vi "反馈节点 1.vi"() -> ()   [LabVIEW 2023]
panel:
  out "compile or load":dbl[](array[numeric])
  out "first call":dbl[](array[numeric])
  out "Array":i32[](array[numeric])
  # "反馈节点 1"
  # "例子 1"
  # "运行 两次以后"
  # "反馈节点 如果初始值 设为 compile or load \n那么 feedback node value will keep last value"
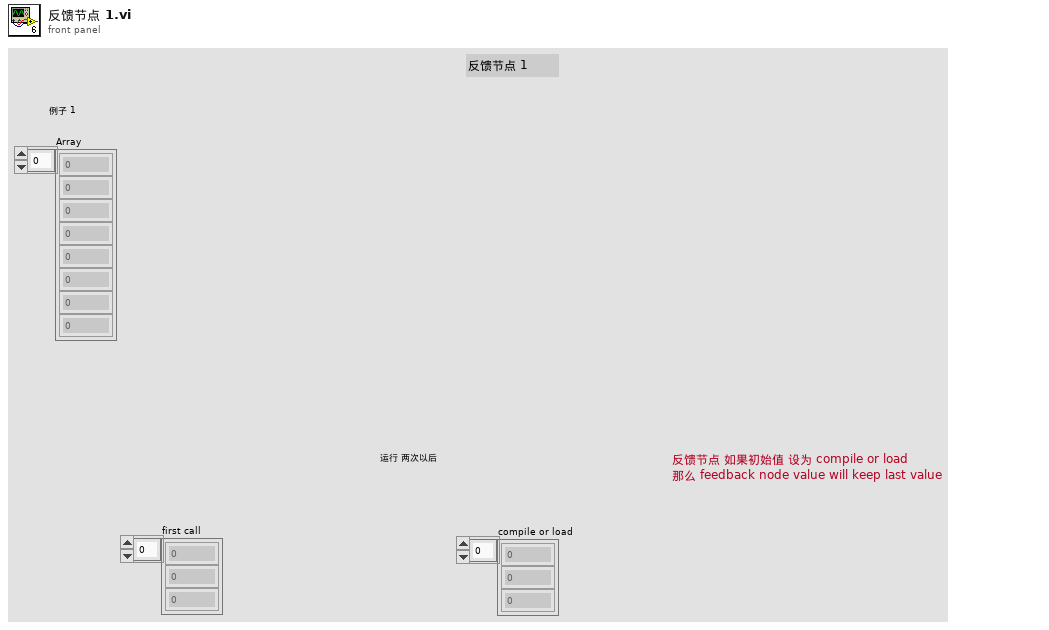
[diagram p1: front panel]
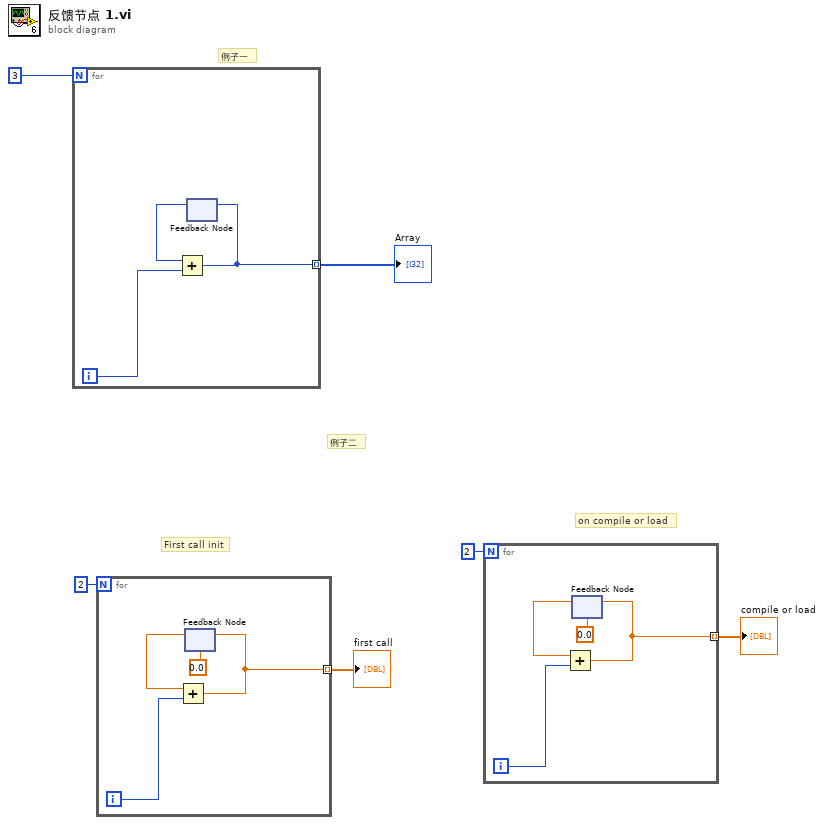
[diagram p0: block diagram]
diagram:
  # "on compile or load"
  # "First call init"
  # "例子二"
  # "例子一"
  n1 = for {
    N: 3 -> [_]
    tunnel: [w7] -> w5 mode=indexing
    i -> [w9]
    n2 = feedback #1() -> (w8:i32)  [unwired: 1 in]
    n3 = Add(x=w8, y=w9) -> (x+y=w7:i32)
    n4 = feedback-in #1(w7) -> ()
  }
  "Array" <- w5
  n5 = for {
    N: 2 -> [_]
    tunnel: [w12] -> w3 mode=indexing
    i -> [w10]
    n6 = feedback #2(0.0) -> (w13:dbl)
    n7 = Add(x=w13, y=w10) -> (x+y=w12:dbl)
    n8 = feedback-in #2(w12) -> ()
  }
  "first call" <- w3
  n9 = for {
    N: 2 -> [_]
    tunnel: [w16] -> w1 mode=indexing
    i -> [w14]
    n10 = feedback #3(0.0) -> (w17:dbl)
    n11 = Add(x=w17, y=w14) -> (x+y=w16:dbl)
    n12 = feedback-in #3(w16) -> ()
  }
  "compile or load" <- w1
